vi "Choreo_TrajectorySwerve_GetInitialPose.vi"(9 "mirrorForRedAlliance":bool, 11 "ChoreoTrajectorySwerve":T4) -> (1 "Exists":bool, 3 "InitialPose":T1={"TRANSLATION"={"X"=0.0, "Y"=0.0}, "ROTATION"={"VALUE"=0.0, "COS"=1.0, "SIN"=0.0}} {"ROTATION"."SIN" format="%13.4f"; "ROTATION"."COS" format="%13.4f"; "ROTATION"."VALUE" format="%13.4f"; "TRANSLATION"."Y" format="%14.3f"; "TRANSLATION"."X" format="%14.3f"})   [LabVIEW 2019, in "ChoreoLib.lvlib"]
doc: "Create an empty trajectory\n\nInputs: \n <none>\n\nOutputs:\n - ChoreoTrajectory - array - Empty array of Trajectory states."
uses:
  ChoreoLib.lvlib
  <vilib>/Rock Robotics/WPI/ThirdParty/JAS_Junk/TrajLib/TypeDef/POSE2D.ctl
  <vilib>/Rock Robotics/WPI/ThirdParty/JAS_Junk/TrajLib/Trajectory_Library.lvlib
  <vilib>/Rock Robotics/WPI/ThirdParty/JAS_Junk/TrajLib/TypeDef/ROTATION2D.ctl
  <vilib>/Rock Robotics/WPI/ThirdParty/JAS_Junk/TrajLib/TypeDef/TRANSLATION2D.ctl
  TypeDef/ChoreoSwerveSample.ctl
  TypeDef/ChoreoEventMarker.ctl
  TypeDef/ChoreoTrajectorySwerve.ctl
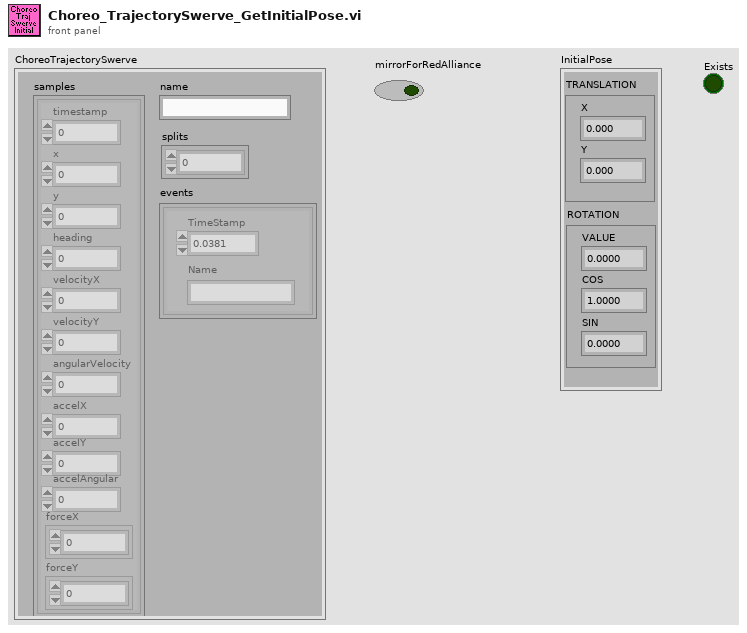
[diagram p1: front panel]
types:
  T1 = typedef "Trajectory_Library.lvlib/POSE2D.ctl" = cluster{"TRANSLATION":T2, "ROTATION":T3}
  T2 = typedef "Trajectory_Library.lvlib/TRANSLATION2D.ctl" = cluster{"X":dbl, "Y":dbl}
  T3 = typedef "Trajectory_Library.lvlib/ROTATION2D.ctl" = cluster{"VALUE":dbl, "COS":dbl, "SIN":dbl}
  T4 = typedef "ChoreoLib.lvlib/ChoreoTrajectorySwerve.ctl" = cluster{"name":string, "samples":T5[], "splits":i32[], "events":T6[]}
  T5 = typedef "ChoreoLib.lvlib/ChoreoSwerveSample.ctl" = cluster{"timestamp":dbl, "x":dbl, "y":dbl, "heading":dbl, "velocityX":dbl, "velocityY":dbl, "angularVelocity":dbl, "accelX":dbl, "accelY":dbl, "accelAngular":dbl, "forceX":dbl[], "forceY":dbl[]}
  T6 = typedef "ChoreoLib.lvlib/ChoreoEventMarker.ctl" = cluster{"TimeStamp":dbl, "Name":string}
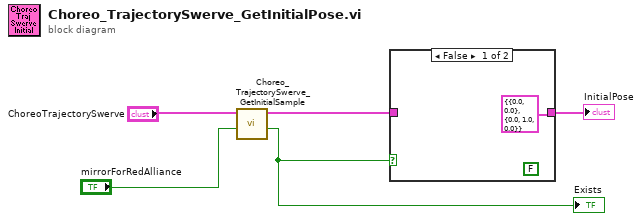
[diagram p0: block diagram]
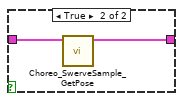
[diagram p2: hidden frame]
diagram:
  n1 = call "Choreo_TrajectorySwerve_GetInitialSample.vi"("mirrorForRedAlliance"="mirrorForRedAlliance", "ChoreoTrajectorySwerve"="ChoreoTrajectorySwerve") -> ("Exists"=w3:bool, "sample"=w2:T5)  [unwired: 8 in]
  "Exists" <- w3
  n2 = case shown="False" w3 {
    tunnel: w2 -> [_ w8]
    tunnel: [T1 {"TRANSLATION"={"X"=0.0, "Y"=0.0}, "ROTATION"={"VALUE"=0.0, "COS"=1.0, "SIN"=0.0}} ("Pose") w7] -> w1
    frame False {
      (unwired) FALSE
    }
    frame True {
      n3 = call "Choreo_SwerveSample_GetPose.vi"("ChoreoSwerveSample"=w8) -> ("Pose"=w7:T1)  [unwired: 10 in]
    }
  }
  "InitialPose" <- w1
